vi "Dashboard Main.vi"() -> ()   [LabVIEW 2011]
uses:
  <vilib>/Rock Robotics/WPI/DriverStation/WPI_DriverStationDigitalData.ctl
  High Priority Dash Data.ctl
panel:
  out "Boolean":bool
  out "8 -- Battery":sgl(graph)
  out "Analog Input":sgl[](array[slide]) scale=0.0..5.0
  in  "Viewer":enum32{"Camera Image", "Kinect Skeleton"}(tab)
  in  "Video Enable":bool=TRUE
  out "Camera Image":T1(plugin-control)
  out "Buttons 1":cluster{"1":bool, "2":bool, "3":bool}
  out "Kinect 1":cluster{"X":dbl, "Y":dbl, "Z":dbl} {"X" scale=1.0..-1.0; "Y" scale=1.0..-1.0; "Z" scale=1.0..-1.0}
  out "Buttons 2":cluster{"1":bool, "2":bool, "3":bool}
  out "Kinect 2":cluster{"X":dbl, "Y":dbl, "Z":dbl} {"X" scale=1.0..-1.0; "Y" scale=1.0..-1.0; "Z" scale=1.0..-1.0}
  out "Version":string
  out "Skeleton Picture":picture
  out "Players":i8
  out "Dashboard Datatype Warning":string="Warning: The Dashboard Datatype used by the robot project and this dashboard do not match.\nSee diagram for more details."
  out "Robot IP Address":string
  out "Image Error Message":string="Timeout in Camera Communications"
  out "Solenoid Output":bool[](array[boolean])
  out "PWM":cluster{u8, u8}[](array[slide])=[{0, 157}, {0, 157}, {0, 157}, {0, 157}, {0, 157}, {0, 157}, {0, 157}, {0, 157}, {0, 157}, {0, 169}] scale=1.0..255.0
  out "GPIO Output Enable":bool[](array[boolean])
  out "GPIO State":bool[](array[boolean])
  out "Relay":cluster{"Forward":bool[], "Reverse":bool[]}
  # "Analog #1"
  # "1"
  # "7"
  # "Communications"
  # "Solenoid #1"
  # "1"
  # "8"
  # "Digital #1"
  # "1"
  # "10"
  # "1"
  # "14"
  # "1"
  # "8"
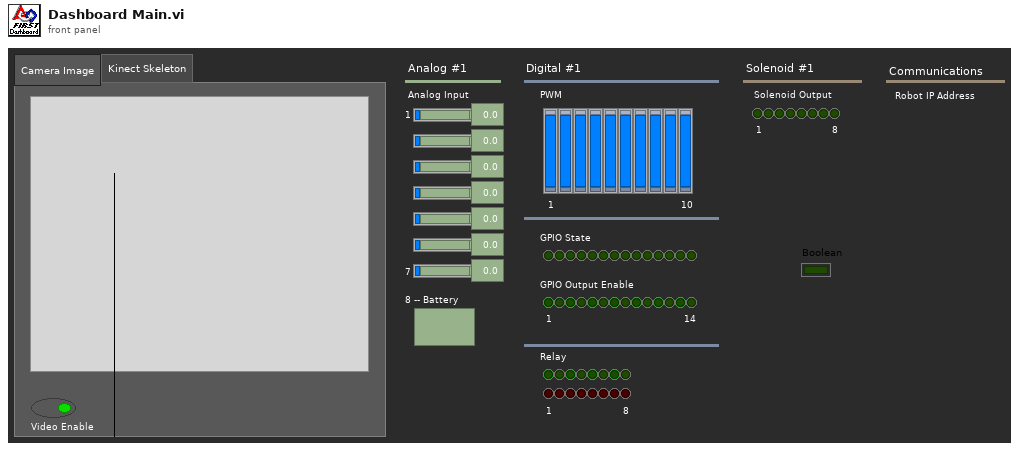
[diagram p1: front panel]
types:
  T1 = typedef "IMAQ Image.ctl" = refnum<image>
  T2 = typedef "High Priority Dash Data.ctl" = cluster{cluster{bool, i32, i32, i32, i32}, cluster{bool, i32, i32, i32, i32}, cluster{bool, i32, i32, i32, i32}, cluster{bool, i32, i32, i32, i32}}
  T3 = typedef "WPI_DriverStationDigitalData.ctl" = cluster{"Relay Fwd":u8, "Relay Rev":u8, "GPIO":u16, "GPIO_OE":u16, "PWM":cluster{"PWM[0]":u8, "PWM[1]":u8, "PWM[2]":u8, "PWM[3]":u8, "PWM[4]":u8, "PWM[5]":u8, "PWM[6]":u8, "PWM[7]":u8, "PWM[8]":u8, "PWM[9]":u8}}
  T4 = cluster{cluster{"AnalogModule[0]":cluster{"Channel[0]":sgl, "Channel[1]":sgl, "Channel[2]":sgl, "Channel[3]":sgl, "Channel[4]":sgl, "Channel[5]":sgl, "Channel[6]":sgl, "Channel[7]":sgl}, "AnalogModule[1]":cluster{"Channel[0]":sgl, "Channel[1]":sgl, "Channel[2]":sgl, "Channel[3]":sgl, "Channel[4]":sgl, "Channel[5]":sgl, "Channel[6]":sgl, "Channel[7]":sgl}}, cluster{"DigitalModule[0]":T3, "DigitalModule[1]":T3}, "Solenoid":u8}
  T5 = typedef "Image Type" = u32
  T6 = cluster{"Competition mode":bool, "Robot Link":bool, "Autonomous":bool, "Enabled":bool, "E-Stop":bool}
  T7 = cluster{"AnalogModule[0]":cluster{"Channel[0]":sgl, "Channel[1]":sgl, "Channel[2]":sgl, "Channel[3]":sgl, "Channel[4]":sgl, "Channel[5]":sgl, "Channel[6]":sgl, "Channel[7]":sgl}, "AnalogModule[1]":cluster{"Channel[0]":sgl, "Channel[1]":sgl, "Channel[2]":sgl, "Channel[3]":sgl, "Channel[4]":sgl, "Channel[5]":sgl, "Channel[6]":sgl, "Channel[7]":sgl}}
  T8 = cluster{"DigitalModule[0]":T3, "DigitalModule[1]":T3}
  T9 = cluster{"Channel[0]":sgl, "Channel[1]":sgl, "Channel[2]":sgl, "Channel[3]":sgl, "Channel[4]":sgl, "Channel[5]":sgl, "Channel[6]":sgl, "Channel[7]":sgl}[]
  T10 = cluster{"Channel[0]":sgl, "Channel[1]":sgl, "Channel[2]":sgl, "Channel[3]":sgl, "Channel[4]":sgl, "Channel[5]":sgl, "Channel[6]":sgl, "Channel[7]":sgl}
  T11 = typedef "LVRectTypeDef.ctl" = cluster{"left":i16, "top":i16, "right":i16, "bottom":i16}
  T12 = typedef "SkeletonTrackState.ctl" = enum32{"NotTracked", "PositionOnly", "Tracked"}
  T13 = cluster{"TrackingState":u8[], "Position":cluster{"x":sgl, "y":sgl, "z":sgl}, cluster{"x":sgl, "y":sgl, "z":sgl, sgl}[], "TrackState":T12}
  T14 = cluster{cluster{"ScaledToPercentRange":dbl, "ScaledToPercentRange":dbl, "ScaledToPercentRange":dbl}, cluster{bool, bool, bool}}[]
  T15 = typedef "LVBoundsTypeDef.ctl" = cluster{"Width":u32, "Height":u32}
  T16 = cluster{cluster{"ScaledToPercentRange":dbl, "ScaledToPercentRange":dbl, "ScaledToPercentRange":dbl}, cluster{bool, bool, bool}}
  T17 = cluster{"ScaledToPercentRange":dbl, "ScaledToPercentRange":dbl, "ScaledToPercentRange":dbl}
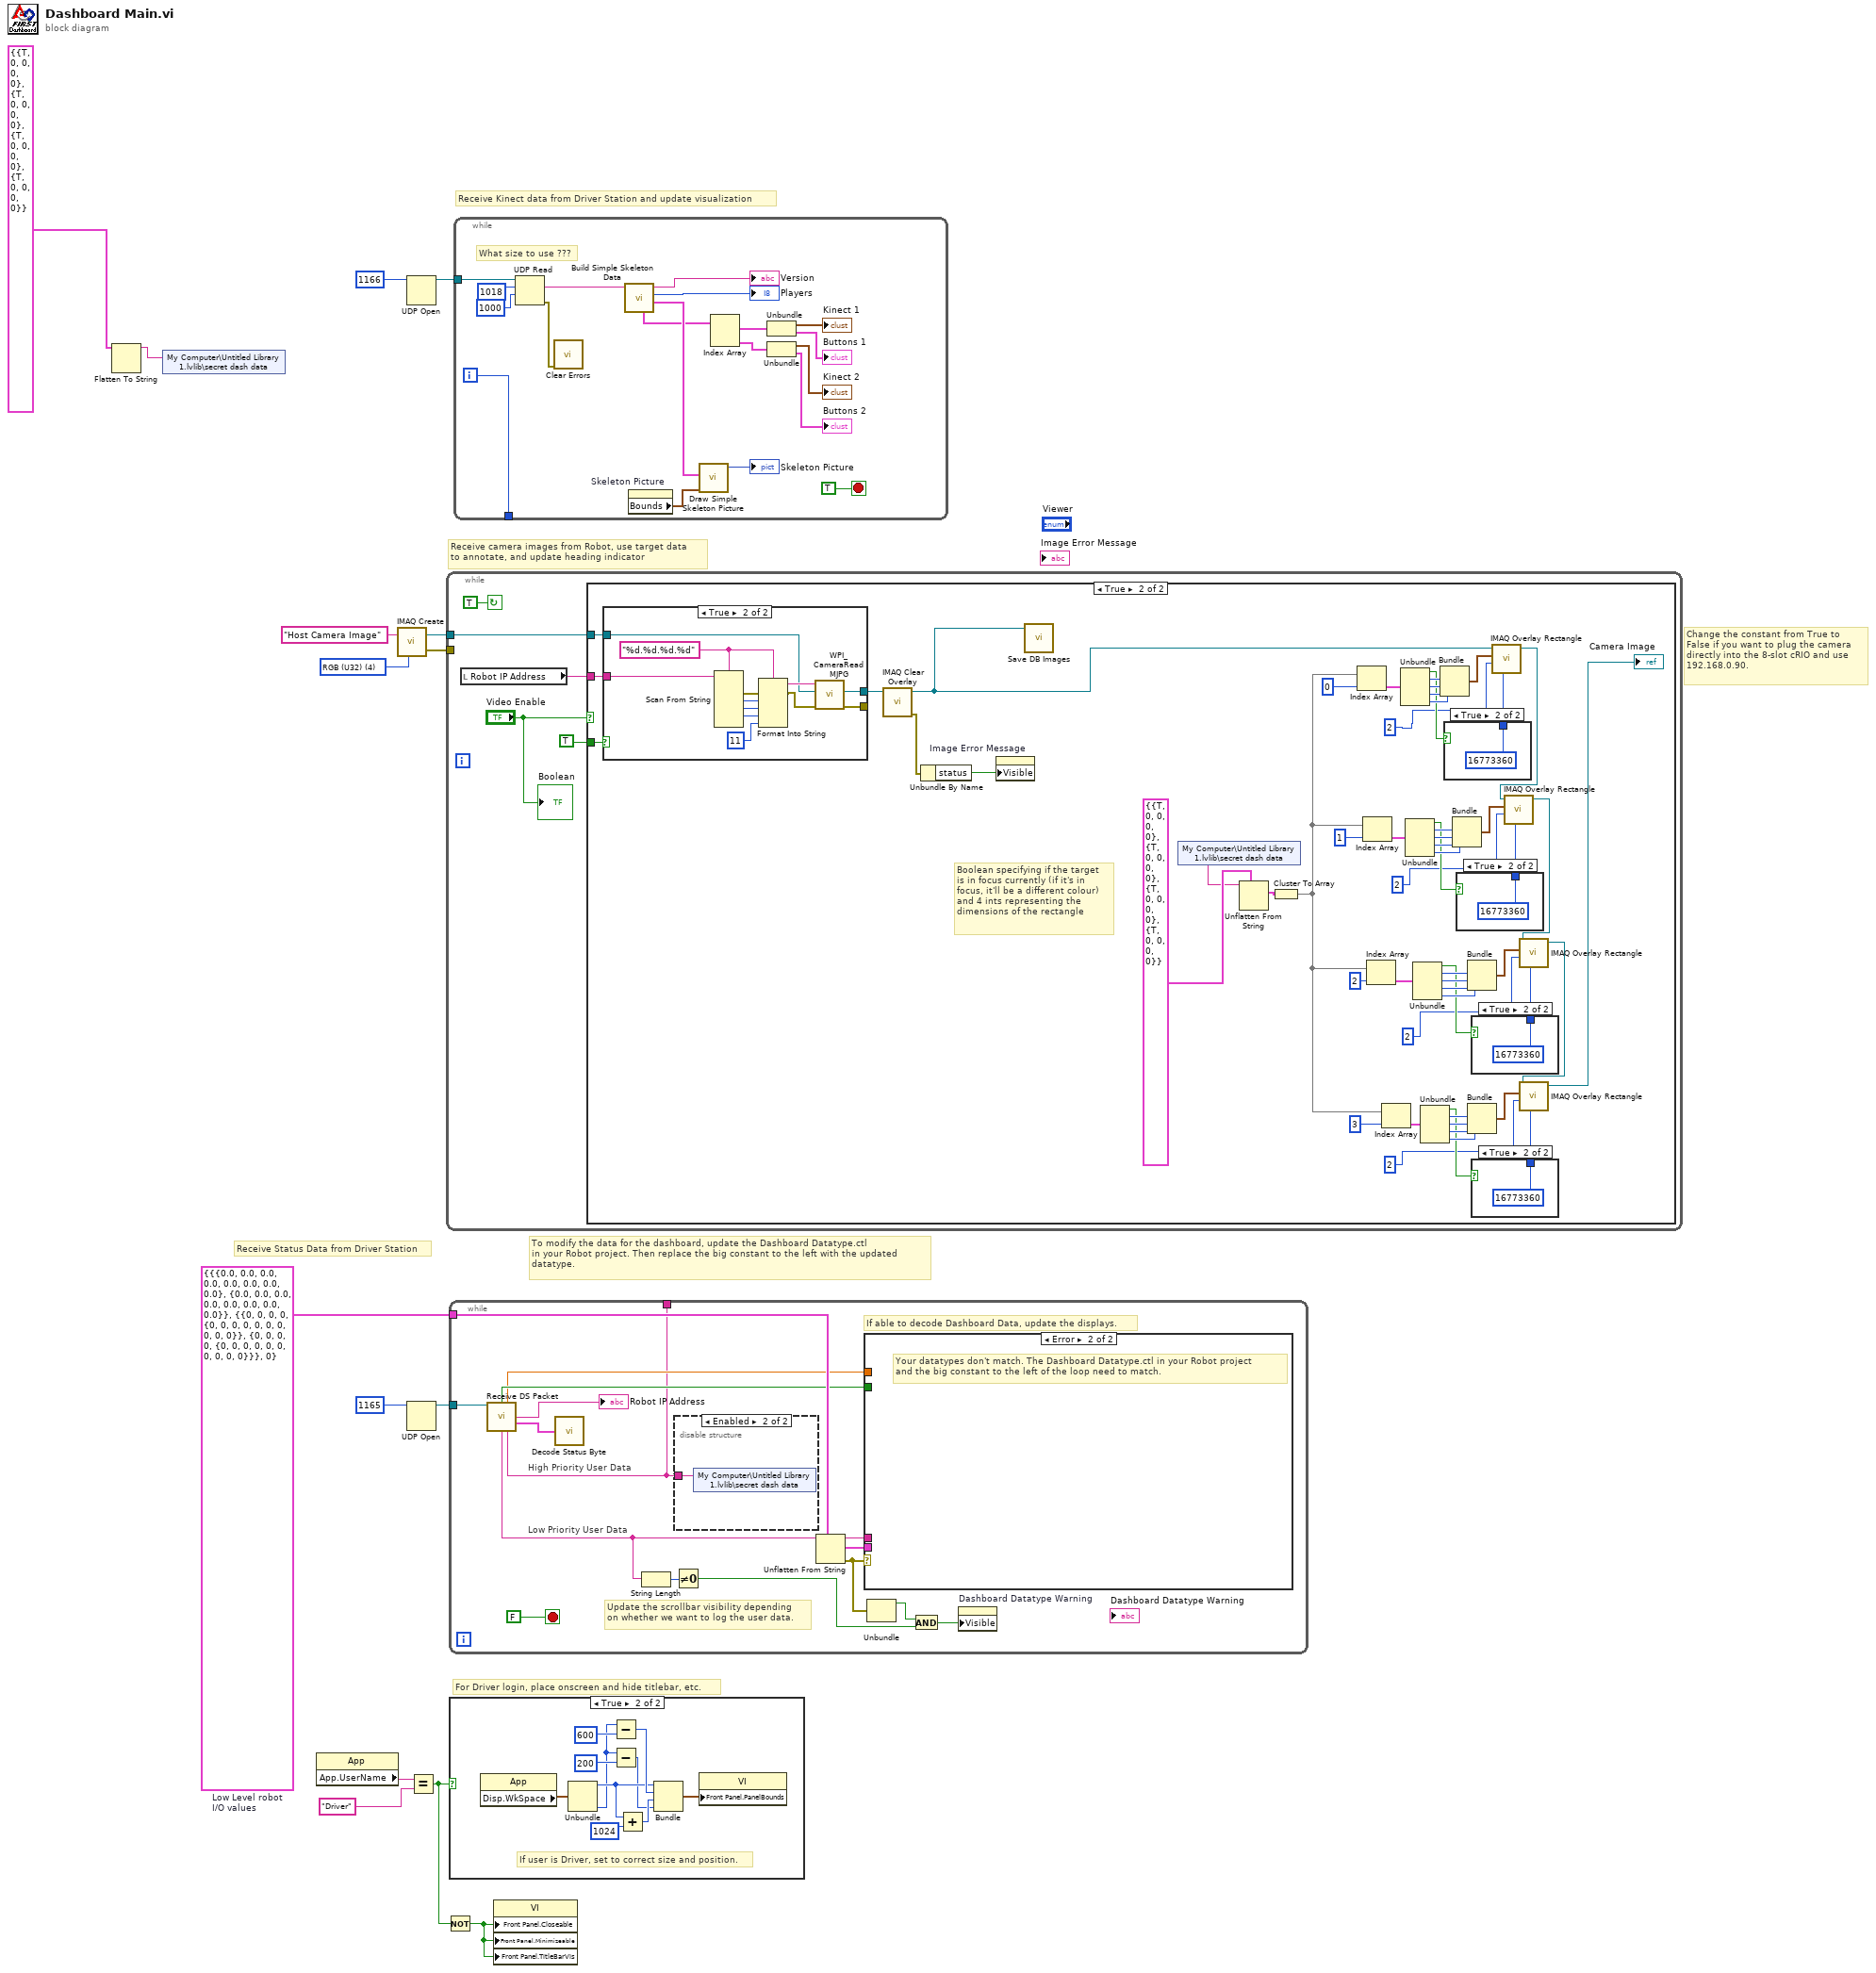
[diagram p0: block diagram]
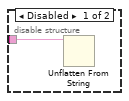
[diagram p3: hidden frame]
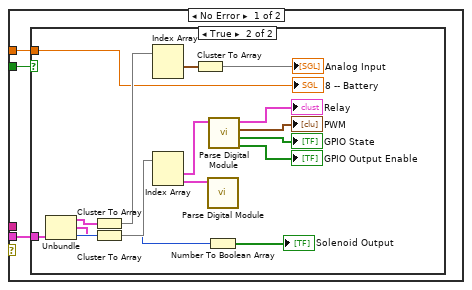
[diagram p4: hidden frame]
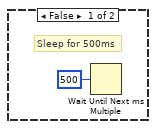
[diagram p6: hidden frame]
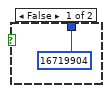
[diagram p7: hidden frame]
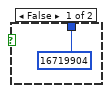
[diagram p8: hidden frame]
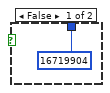
[diagram p9: hidden frame]
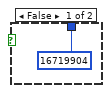
[diagram p10: hidden frame]
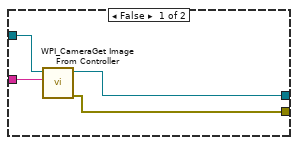
[diagram p11: hidden frame]
diagram:
  w5 = T4 {{"AnalogModule[0]"={"Channel[0]"=0.0, "Channel[1]"=0.0, "Channel[2]"=0.0, "Channel[3]"=0.0, "Channel[4]"=0.0, "Channel[5]"=0.0, "Channel[6]"=0.0, "Channel[7]"=0.0}, "AnalogModule[1]"={"Channel[0]"=0.0, "Channel[1]"=0.0, "Channel[2]"=0.0, "Channel[3]"=0.0, "Channel[4]"=0.0, "Channel[5]"=0.0, "Channel[6]"=0.0, "Channel[7]"=0.0}}, {"DigitalModule[0]"={"Relay Fwd"=0, "Relay Rev"=0, "GPIO"=0, "GPIO_OE"=0, "PWM"={"PWM[0]"=0, "PWM[1]"=0, "PWM[2]"=0, "PWM[3]"=0, "PWM[4]"=0, "PWM[5]"=0, "PWM[6]"=0, "PWM[7]"=0, "PWM[8]"=0, "PWM[9]"=0}}, "DigitalModule[1]"={"Relay Fwd"=0, "Relay Rev"=0, "GPIO"=0, "GPIO_OE"=0, "PWM"={"PWM[0]"=0, "PWM[1]"=0, "PWM[2]"=0, "PWM[3]"=0, "PWM[4]"=0, "PWM[5]"=0, "PWM[6]"=0, "PWM[7]"=0, "PWM[8]"=0, "PWM[9]"=0}}}, "Solenoid"=0}  # Low Level robot I/O values
  w13 = T5 4 items=["Grayscale (U8)", "Grayscale (I16)", "Grayscale (SGL)", "Complex (CSG)", "RGB (U32)", "HSL (U32)", "RGB (U64)"] ("Image Type")
  # "Change the constant from True to\nFalse if you want to plug the camera\ndirectly into the 8-slot cRIO and use\n192.168.0.90."
  # "Receive Kinect data from Driver Station and update visualization"
  # "For Driver login, place onscreen and hide titlebar, etc."
  # "To modify the data for the dashboard, update the Dashboard Datatype.ctl\nin your Robot project. Then replace the big constant to the left with the updated\ndatatype."
  # "Receive Status Data from Driver Station"
  # "Receive camera images from Robot, use target data\nto annotate, and update heading indicator"
  n1 = Flatten To String(anything=T2 {{TRUE, 0, 0, 0, 0}, {TRUE, 0, 0, 0, 0}, {TRUE, 0, 0, 0, 0}, {TRUE, 0, 0, 0, 0}}) -> (data string=w2:string)  [unwired: 3 in, 2 out]
  n2 = shared-variable "My Computer\\Untitled Library 1.lvlib\\secret dash data"(w2) -> ()  [unwired: 1 in, 1 out]
  n3 = property class="App"() -> ("App.UserName"=w8:string)  [unwired: 2 in, 2 out]
  n4 = call "IMAQ Create"("Image Name"="Host Camera Image", "Image Type"=w13) -> ("New Image"=w11:T1, "error out"=w10:errorcluster)  [unwired: 2 in, 1 out]
  n5 = UDP Open(11:u16 1166 ("port")) -> (port=w3:refnum<k16>)  [unwired: 2 in, 4 out]
  n6 = UDP Open(11:u16 1165 ("port")) -> (port=w14:refnum<k16>)  [unwired: 2 in, 4 out]
  n7 = Equal?(x=w8, y="Driver") -> (x = y?=w7:bool)
  n8 = Not(x=w7) -> (.not. x?=w6:bool)
  n9 = while {
    tunnel: w11 -> [w18]
    tunnel: w10 -> [_]
    stop <- TRUE continue-if-true
    n10 = local read "Robot IP Address"() -> (w19:string)
    n11 = case shown="True" "Video Enable" {
      tunnel: w19 -> [_ w76]
      tunnel: w18 -> [_ w75]
      tunnel: TRUE -> [_ w71]
      frame False {
        # "Sleep for 500ms"
        n12 = Wait Until Next ms Multiple(millisecond multiple=u32 500) -> ()  [unwired: 1 out]
      }
      frame True {
        # "Boolean specifying if the target\nis in focus currently (if it's in \nfocus, it'll be a different colour)\nand 4 ints representing the\ndimensions of the rectangle"
        n13 = case shown="True" w71 {
          tunnel: w75 -> [w87 w94]
          tunnel: [w85 w92] -> _
          tunnel: [w86 w93] -> w72
          tunnel: w76 -> [w88 w97]
          frame False {
            n14 = call <vilib>:"WPI_CameraGet Image From Controller.vi"("Controller Address"=w88, "Image"=w87) -> ("error out"=w85:errorcluster, "Image Out"=w86:T1)  [unwired: 2 in, 6 out]
          }
          frame True {
            w89 = "%d.%d.%d.%d" ("format string")
            n15 = Scan From String(format string=w89, input string=w97) -> (error out=w96:errorcluster, output 1=w98:i32, output 2=w99:i32, output 3=w100:i32)  [unwired: 2 in, 7 out]
            n16 = Format Into String(format string=w89, error in=w96, w98, w99, w100, 11 ("IP Suffix:")) -> (resulting string=w95:string, error out=w91:errorcluster)  [unwired: 1 in]
            n17 = call <vilib>:"WPI_CameraRead MJPG.vi"("error in"=w91, "Image"=w94, "address"=w95) -> ("error out"=w92:errorcluster, "Image Out"=w93:T1)  [unwired: 7 in]
          }
        }
        n18 = call "IMAQ Clear Overlay"("Image"=w72) -> ("error out"=w73:errorcluster, "Image Out"=w22:T1)  [unwired: 2 in, 7 out]
        n19 = Unbundle By Name(w73) -> ("status"=w74:bool)
        n20 = property on="Image Error Message" class="Str"("Visible"=w74) -> ()  [unwired: 2 in, 2 out]
        n21 = call "Save DB Images.vi"("Image"=w22) -> ()  [unwired: 2 in, 1 out]
        n22 = shared-variable "My Computer\\Untitled Library 1.lvlib\\secret dash data"() -> (w27:string)  [unwired: 1 in, 1 out]
        n23 = Unflatten From String(type=T2 {{TRUE, 0, 0, 0, 0}, {TRUE, 0, 0, 0, 0}, {TRUE, 0, 0, 0, 0}, {TRUE, 0, 0, 0, 0}}, binary string=w27) -> (value=w62:T2)  [unwired: 1 in, 4 out]
        n24 = Cluster To Array(cluster=w62) -> (array=w32:cluster{bool, i32, i32, i32, i32}[])
        n25 = Index Array(array=w32, index=0) -> (element=w60:cluster{bool, i32, i32, i32, i32})
        n26 = Index Array(array=w32, index=1) -> (element=w51:cluster{bool, i32, i32, i32, i32})
        n27 = Index Array(array=w32, index=2) -> (element=w42:cluster{bool, i32, i32, i32, i32})
        n28 = Index Array(array=w32, index=3) -> (element=w33:cluster{bool, i32, i32, i32, i32})
        n29 = Unbundle(w60) -> (w63:bool, w64:i32, w65:i32, w67:i32, w66:i32)
        n30 = Unbundle(w51) -> (w53:bool, w54:i32, w55:i32, w57:i32, w56:i32)
        n31 = Unbundle(w42) -> (w44:bool, w45:i32, w46:i32, w48:i32, w47:i32)
        n32 = Unbundle(w33) -> (w35:bool, w36:i32, w37:i32, w39:i32, w38:i32)
        n33 = Bundle(w64, w65, w67, w66) -> (w69:cluster{i32, i32, i32, i32})  [unwired: 1 in]
        n34 = case shown="True" w63 {
          tunnel: [16719904 16773360] -> w68
          frame False {
          }
          frame True {
          }
        }
        n35 = Bundle(w54, w55, w57, w56) -> (w59:cluster{i32, i32, i32, i32})  [unwired: 1 in]
        n36 = case shown="True" w53 {
          tunnel: [16719904 16773360] -> w58
          frame False {
          }
          frame True {
          }
        }
        n37 = Bundle(w45, w46, w48, w47) -> (w50:cluster{i32, i32, i32, i32})  [unwired: 1 in]
        n38 = Bundle(w36, w37, w39, w38) -> (w41:cluster{i32, i32, i32, i32})  [unwired: 1 in]
        n39 = case shown="True" w44 {
          tunnel: [16719904 16773360] -> w49
          frame False {
          }
          frame True {
          }
        }
        n40 = case shown="True" w35 {
          tunnel: [16719904 16773360] -> w40
          frame False {
          }
          frame True {
          }
        }
        n41 = call "IMAQ Overlay Rectangle"("Color"=w68, "Drawing Mode (Frame)"=2, "Rectangle"=w69, "Image"=w22) -> ("Image Out"=w31:T1)  [unwired: 6 in, 1 out]
        n42 = call "IMAQ Overlay Rectangle"("Color"=w58, "Drawing Mode (Frame)"=2, "Rectangle"=w59, "Image"=w31) -> ("Image Out"=w30:T1)  [unwired: 6 in, 1 out]
        n43 = call "IMAQ Overlay Rectangle"("Color"=w49, "Drawing Mode (Frame)"=2, "Rectangle"=w50, "Image"=w30) -> ("Image Out"=w29:T1)  [unwired: 6 in, 1 out]
        n44 = call "IMAQ Overlay Rectangle"("Color"=w40, "Drawing Mode (Frame)"=2, "Rectangle"=w41, "Image"=w29) -> ("Image Out"=→"Camera Image":T1)  [unwired: 6 in, 1 out]
      }
    }
    "Boolean" <- "Video Enable"
  }
  n45 = while {
    tunnel: w14 -> [w114]
    tunnel: w5 -> [w113]
    tunnel: [w101] -> _
    stop <- FALSE stop-if-true
    # "High Priority User Data"
    # "Low Priority User Data"
    # "Update the scrollbar visibility depending\non whether we want to log the user data."
    # "If able to decode Dashboard Data, update the displays."
    n46 = call "Receive DS Packet.vi"("Recv Socket"=w114) -> ("New Dashboard Data"=w110:bool, "Battery"=w102:sgl, "Robot IP Address"=→"Robot IP Address":string, "Status"=w115:T6, "Low Priority User Data"=w103:string, "High Priority User Data"=w101:string)  [unwired: 1 in, 8 out]
    n47 = call "Decode Status Byte.vi"("Status Byte"=w115) -> ()  [unwired: 2 out]
    n48 = String Length(string=w103) -> (length=w105:i32)
    n49 = Not Equal To 0?(x=w105) -> (x != 0?=w108:bool)
    n50 = disable-structure shown="Enabled" {
      disable-tunnel: w101 -> [w117 w118]
      frame Disabled {
        n51 = Unflatten From String(binary string=w117) -> ()  [unwired: 2 in, 5 out]
      }
      frame Enabled {
        n52 = shared-variable "My Computer\\Untitled Library 1.lvlib\\secret dash data"(w118) -> ()  [unwired: 1 in, 1 out]
      }
    }
    n53 = Unflatten From String(type=w113, binary string=w103) -> (rest of the binary string=w106:string, value=w112:T4, error out=w111:errorcluster)  [unwired: 1 in, 2 out]
    n54 = case shown="Error" w111 {
      tunnel: w112 -> [w121 _]
      tunnel: w110 -> [w120 _]
      tunnel: w106 -> [_ _]
      tunnel: w102 -> [w119 _]
      frame No Error {
        n55 = case shown="True" w120 {
          tunnel: w121 -> [_ w128]
          tunnel: w119 -> [_ w122]
          frame False {
            # "Don't update if the robot hasn't sent new data"
          }
          frame True {
            n56 = Unbundle(w128) -> (w125:T7, w126:T8, "Solenoid"=w127:u8)
            n57 = Cluster To Array(cluster=w125) -> (array=w136:T9)
            n58 = Cluster To Array(cluster=w126) -> (array=w135:T3[])
            n59 = Index Array(array=w136) -> (element #1=w123:T10)  [unwired: 2 in, 1 out]
            n60 = Index Array(array=w135) -> (element #1=w134:T3, element #2=w129:T3)  [unwired: 2 in]
            n61 = Cluster To Array(cluster=w123) -> (array=→"Analog Input":sgl[])
            n62 = call "Parse Digital Module.vi"("DigitalModule"=w129) -> ()  [unwired: 11 out]
            n63 = Number To Boolean Array(number=w127) -> (Boolean array=→"Solenoid Output":bool[])
            n64 = call "Parse Digital Module.vi"("DigitalModule"=w134) -> ("GPIO Output Enable"=→"GPIO Output Enable":bool[], "GPIO State"=→"GPIO State":bool[], "PWM"=→"PWM":cluster{u8, u8}[], "Relay"=→"Relay":cluster{"Forward":bool[], "Reverse":bool[]})  [unwired: 7 out]
            "8 -- Battery" <- w122
          }
        }
      }
      frame Error {
        # "Your datatypes don't match. The Dashboard Datatype.ctl in your Robot project\nand the big constant to the left of the loop need to match."
      }
    }
    n65 = Unbundle(w111) -> ("status"=w107:bool)  [unwired: 2 out]
    n66 = And(x=w107, y=w108) -> (x .and. y?=w109:bool)
    n67 = property on="Dashboard Datatype Warning" class="Str"("Visible"=w109) -> ()  [unwired: 2 in, 2 out]
  }
  n68 = case shown="True" w7 {
    frame False {
    }
    frame True {
      # "If user is Driver, set to correct size and position."
      n69 = property class="App"() -> ("Disp.WkSpace"=w147:T11)  [unwired: 2 in, 2 out]
      n70 = Unbundle(w147) -> ("left"=w142:i16, "bottom"=w138:i16)  [unwired: 2 out]
      n71 = Subtract(x=w138, y=600) -> (x-y=w144:i32)
      n72 = Subtract(x=w138, y=200) -> (x-y=w139:i32)
      n73 = Add(x=w142, y=1024) -> (x+y=w143:i32)
      n74 = Bundle("left"=w142, w144, w143, w139) -> (w146:cluster{"left":i16, i32, i32, i32})  [unwired: 1 out]
      n75 = property class="VI"("Front Panel.PanelBounds"=w146) -> ()  [unwired: 2 in, 2 out]
    }
  }
  n76 = while {
    tunnel: w3 -> [w164]
    tunnel: [w148] -> _
    i -> [w148]
    stop <- TRUE stop-if-true
    # "What size to use ???"
    n77 = UDP Read(connection ID=w164, max size (548)=1018 ("bytes to read"), timeout ms (25000)=1000) -> (data out=w158:string, error out=w156:errorcluster)  [unwired: 1 in, 3 out]
    n78 = call <vilib>:"Clear Errors.vi"("error in (no error)"=w156) -> ()  [unwired: 6 in, 1 out]
    n79 = call "Build Simple Skeleton Data.vi"("data out"=w158) -> ("Skeleton Data"=w159:T13, "NumPlayers"=→"Players":i8, "Version String"=→"Version":string, "Simple Joystick Info"=w155:T14)  [unwired: 6 in, 1 out]
    n80 = property on="Skeleton Picture" class="Pict"() -> ("Bounds"=w160:T15)  [unwired: 2 in, 2 out]
    n81 = call "Draw Simple Skeleton Picture.vi"("Bounds"=w160, "Simple Skeleton"=w159) -> ("new picture out"=→"Skeleton Picture":picture)  [unwired: 9 in]
    n82 = Index Array(array=w155) -> (element #1=w154:T16, element #2=w153:T16)  [unwired: 2 in]
    n83 = Unbundle(w154) -> (→"Kinect 1":T17, →"Buttons 1":cluster{bool, bool, bool})
    n84 = Unbundle(w153) -> (→"Kinect 2":T17, →"Buttons 2":cluster{bool, bool, bool})
  }
  n85 = property class="VI"("Front Panel.Closeable"=w6, "Front Panel.Minimizeable"=w6, "Front Panel.TitleBarVis"=w6) -> ()  [unwired: 2 in, 2 out]
